vi "MGI Bezier Find k Backwards (SGL).vi"(1 "y":sgl format="%.2f", 2 "first k":i32=1, 3 "Bezier Control Points[]":sgl[](array[numeric]) format="%_6g") -> (0 "correct k":i32)   [LabVIEW 2020]
doc: "Search the Bezier Control Points array for the block containing y. y is tested against y(first k - 4*n), where n = 0, 1, .... Return value is (first k - 4*n), suitable for input to Bezier Inverse.\n\nAuthored by David A. Moore\nsupport@mooregoodideas.com\nwww.mooregoodideas.com\n\nCopyright (c) 2010, Moore Good Ideas, Inc.\n\nAll rights reserved.\n\nRedistribution and use in source and binary forms, with or without modification, are permitted provided that the following conditions are met:\n\n * Redistributions of source code must retain the above copyright notice, this list of conditions and the following disclaimer.\n * Redistributions in binary form must reproduce the above copyright notice, this list of conditions and the following disclaimer in the documentation and/or other materials provided with the distribution.\n * Neither the name of Moore Good Ideas, Inc. nor the names of its contributors may be used to endorse or promote products derived from this software without specific prior written permission.\n\nTHIS SOFTWARE IS PROVIDED BY THE COPYRIGHT HOLDERS AND CONTRIBUTORS \"AS IS\" AND ANY EXPRESS OR IMPLIED WARRANTIES, INCLUDING, BUT NOT LIMITED TO, THE IMPLIED WARRANTIES OF MERCHANTABILITY AND FITNESS FOR A PARTICULAR PURPOSE ARE DISCLAIMED. IN NO EVENT SHALL THE COPYRIGHT OWNER OR CONTRIBUTORS BE LIABLE FOR ANY DIRECT, INDIRECT, INCIDENTAL, SPECIAL, EXEMPLARY, OR CONSEQUENTIAL DAMAGES (INCLUDING, BUT NOT LIMITED TO, PROCUREMENT OF SUBSTITUTE GOODS OR SERVICES; LOSS OF USE, DATA, OR PROFITS; OR BUSINESS INTERRUPTION) HOWEVER CAUSED AND ON ANY THEORY OF LIABILITY, WHETHER IN CONTRACT, STRICT LIABILITY, OR TORT (INCLUDING NEGLIGENCE OR OTHERWISE) ARISING IN ANY WAY OUT OF THE USE OF THIS SOFTWARE, EVEN IF ADVISED OF THE POSSIBILITY OF SUCH DAMAGE."
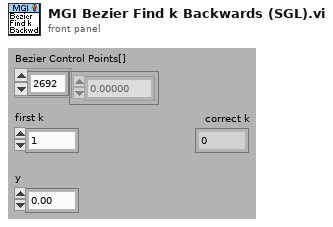
[diagram p1: front panel]
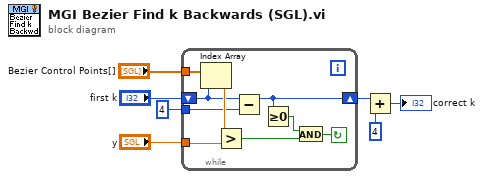
[diagram p0: block diagram]
diagram:
  n1 = while {
    tunnel: "Bezier Control Points[]" -> [w16]
    tunnel: "y" -> [w14]
    shift-right: [w9] -> w4
    shift-left: "first k" -> [w10]
    tunnel: 4 -> [w13]
    stop <- w11 continue-if-true
    n2 = Index Array(array=w16, index=w10) -> (element=w15:sgl)
    n3 = Greater?(x=w15, y=w14) -> (0:w12:bool)
    n4 = Subtract(x=w10, y=w13) -> (x-y=w9:i32)
    n5 = Greater Or Equal To 0?(x=w9) -> (x >= 0?=w8:bool)
    n6 = And(x=w8, y=w12) -> (x .and. y?=w11:bool)
  }
  n7 = Add(x=w4, y=4) -> (x+y=→"correct k":i32)
